vi "gds_rx_close.vi"(8 "error in":errorcluster, 10 "HW parameters":T1={"Device IP Address"="192.168.11.6", "Active Antenna"="RX1", "Carrier Frequency (Hz)"=915000000.0, "Gain (dB)"=10.0, "Trigger Level"=0.01, "Bandwidth (Hz)"=40000000.0, "Reference Position (%)"=10.0, "Capture Time (s)"=0.0004, "Simulate"=FALSE} {"Capture Time (s)" format="%.2p"; "Bandwidth (Hz)" format="%.2p"; "Trigger Level" format="%#.3p"; "Gain (dB)" format="%.2f"; "Carrier Frequency (Hz)" format="%.2p"}) -> (0 "error out":errorcluster)   [LabVIEW 2012]
uses:
  EE 497/LABS/SDR/control_type_defs.llb/rx_hw params.ctl
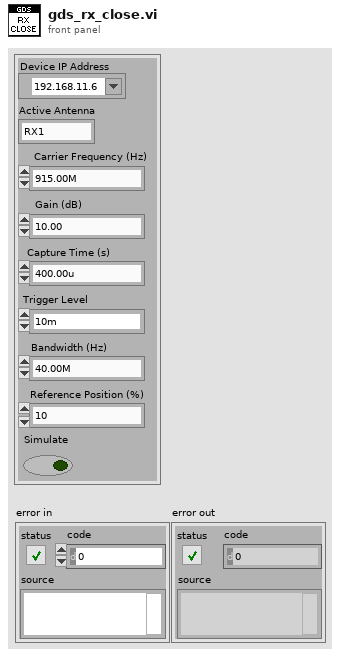
[diagram p1: front panel]
types:
  T1 = typedef "rx_hw params.ctl" = cluster{"Device IP Address":refnum<k15>, "Active Antenna":string, "Carrier Frequency (Hz)":dbl, "Gain (dB)":dbl, "Trigger Level":dbl, "Bandwidth (Hz)":dbl, "Reference Position (%)":dbl, "Capture Time (s)":dbl, "Simulate":bool}
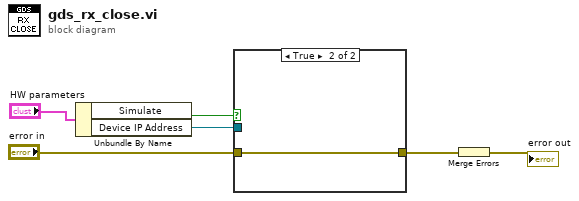
[diagram p0: block diagram]
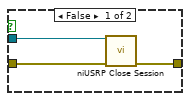
[diagram p2: hidden frame]
diagram:
  n1 = Unbundle By Name("HW parameters") -> ("Simulate"=w5:bool, "Device IP Address"=w4:refnum<k15>)
  n2 = case shown="True" w5 {
    tunnel: w4 -> [w9 _]
    tunnel: "error in" -> [w8 w10]
    tunnel: [w7 w10] -> w3
    frame False {
      n3 = call <instrlib>:"niUSRP Close Session.vi"("session handle"=w9, "error in (no error)"=w8) -> ("error out"=w7:errorcluster)  [unwired: 13 in]
    }
    frame True {
    }
  }
  n4 = Merge Errors(w3) -> (→"error out":errorcluster)
